vi "_scriptGenerateTermSpecs.vi"(0 "Terminal":bool, 1 "Terms[]":refnum<vi>[](array[refnum]), 2 "TermOnlyTermSpecs":T1[](array[typedef]), 3 "index":i32, 4 "terminalDef":T1, 5 "CompleteTermSpecs":T1[](array[typedef]), 8 "replace":bool) -> (6 "TermOnlyTermSpecsOut":T1[](array[typedef]), 7 "CompleteTermSpecsOut":T1[](array[typedef]))   [LabVIEW 2020]
uses:
  <vilib>/Platform/storage/lvStorage.llb/TerminalDef.ctl
  <vilib>/Platform/storage/lvStorage.llb/_TerminalStyle.ctl
  <vilib>/Utility/XNodeSupport.llb/XRect32.ctl
  <vilib>/Platform/storage/lvStorage.llb/_terminalNames.ctl
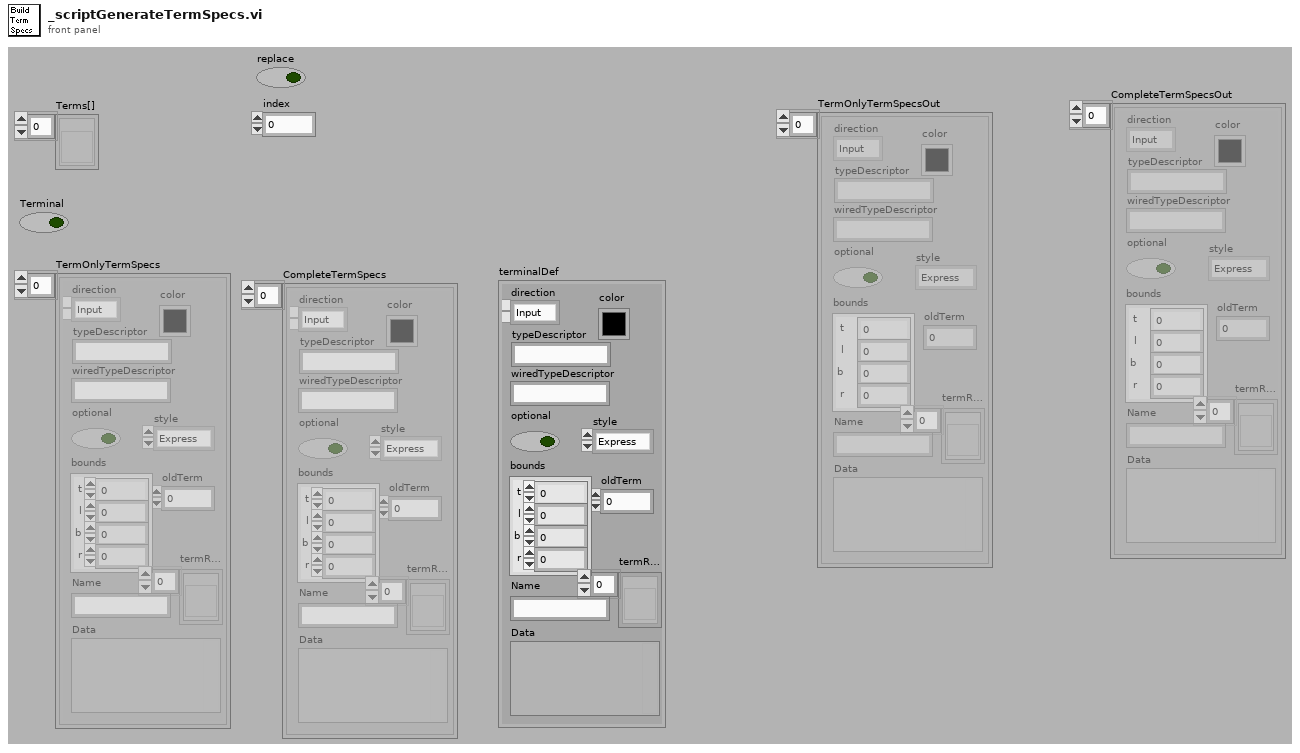
[diagram p1: front panel]
types:
  T1 = typedef "TerminalDef.ctl" = cluster{"direction":enum16{"Input", "Output"}, "typeDescriptor":string, "color":u32, "oldTerm":i32, "style":T2, "optional":bool, "bounds":T3, "termRefs":refnum<vi>[], "Name":string, "Data":variant, "wiredTypeDescriptor":string}
  T2 = typedef "_TerminalStyle.ctl" = enum16{"Express", "Collapsed", "Internal"}
  T3 = typedef "XRect32.ctl" = cluster{"t":i32, "l":i32, "b":i32, "r":i32}
  T4 = typedef "_terminalNames.ctl" = enum16{"Data object in", "Data object out", "PropertyName", "Value", "error in", "error out", "error in (no error)", "Enum strings", "Property name", "Parent object in", "Parent object out", "Object type", "Child object", "Name", "Channel name", "Waveform in", "Data Object", "Data storage in", "Data storage out", "Comparison operator", "Query expression", "Child objects only", "Data objects", "Values", "Signal", "append / replace", "index", "count"}
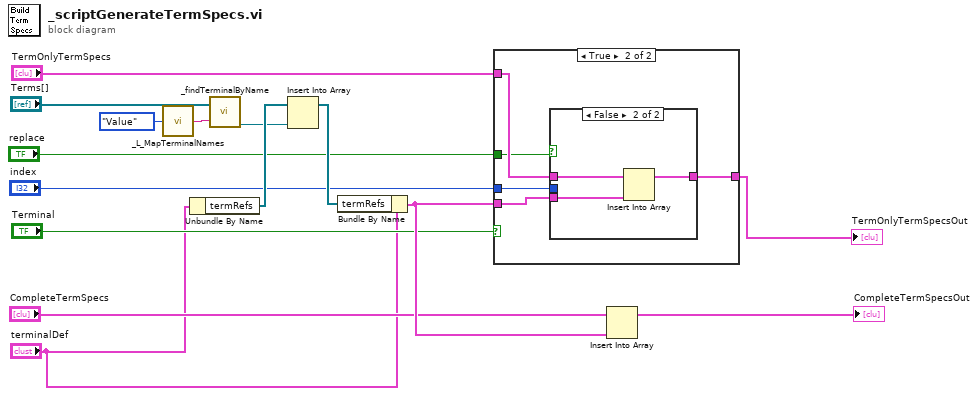
[diagram p0: block diagram]
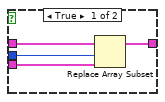
[diagram p3: hidden frame]
diagram:
  n1 = call <vilib>:"_L_MapTerminalNames.vi"("DNL_terminal_in"=_terminalNames."Value") -> ("DNL_name_out"=w11:string)
  n2 = Unbundle By Name("terminalDef") -> ("termRefs"=w14:refnum<vi>[])
  n3 = call <vilib>:"_findTerminalByName.vi"("element"=w11, "Terms[]"="Terms[]") -> ("Term Refnum"=w12:refnum<vi>)  [unwired: 1 out]
  n4 = Insert Into Array(array=w14, new element=w12) -> (w13:refnum<vi>[])  [unwired: 1 in]
  n5 = Bundle By Name(cluster="terminalDef", "termRefs"=w13) -> (w15:T1)
  n6 = case shown="True" "Terminal" {
    tunnel: "TermOnlyTermSpecs" -> [w16 w21]
    tunnel: [w16 w20] -> w4
    tunnel: w15 -> [_ w19]
    tunnel: "replace" -> [_ w18]
    tunnel: "index" -> [_ w17]
    frame False {
    }
    frame True {
      n7 = case shown="False" w18 {
        tunnel: w21 -> [w25 w28]
        tunnel: w19 -> [w24 w27]
        tunnel: [w23 w26] -> w20
        tunnel: w17 -> [w22 _]
        frame True {
          n8 = Replace Array Subset(array=w25, new element=w24, index=w22) -> (w23:T1[])
        }
        frame False {
          n9 = Insert Into Array(array=w28, new element=w27) -> (w26:T1[])  [unwired: 1 in]
        }
      }
    }
  }
  "TermOnlyTermSpecsOut" <- w4
  n10 = Insert Into Array(array="CompleteTermSpecs", new element=w15) -> (→"CompleteTermSpecsOut":T1[])  [unwired: 1 in]
